vi "Main.vi"() -> ()   [LabVIEW 2018, in "Main.lvlib"]
uses:
  Main.lvlib
  database/Items--cluster.ctl
  database/Purchased_Items--cluster.ctl
  database/Visits--cluster.ctl
  image management/Image Management.lvlib
  receipt parsing/Receipt Parsing.lvlib
  database/Database.lvlib
panel:
  out "Timestamp":timestamp[](array[timestamp])
  out "TotalPrice":dbl
  out "Unit":string[](array[string])
  out "NumberOfUnits":dbl[](array[numeric])
  out "TaxStatus":string[](array[string])
  out "PrintedNames":string[](array[string])
  out "Prices":string[](array[string])
  out "Items":string[](array[string])
  out "Footer":string[](array[string])
  out "Header":string[](array[string])
  out "Main Body":string[](array[string])
  out "Image 2":T1(plugin-control)
  out "Array":string[](array[string])
  out "Columns (Pixels)":i32
  out "Rows (Pixels)":i32
  out "Image":T1(plugin-control)
  out "Rows Where Whitespace Starts":i32[](array[numeric])
  out "Image Pixels (I16)":i16[][](array[numeric])
  out "Error Out":errorcluster
  in  "Error In":errorcluster
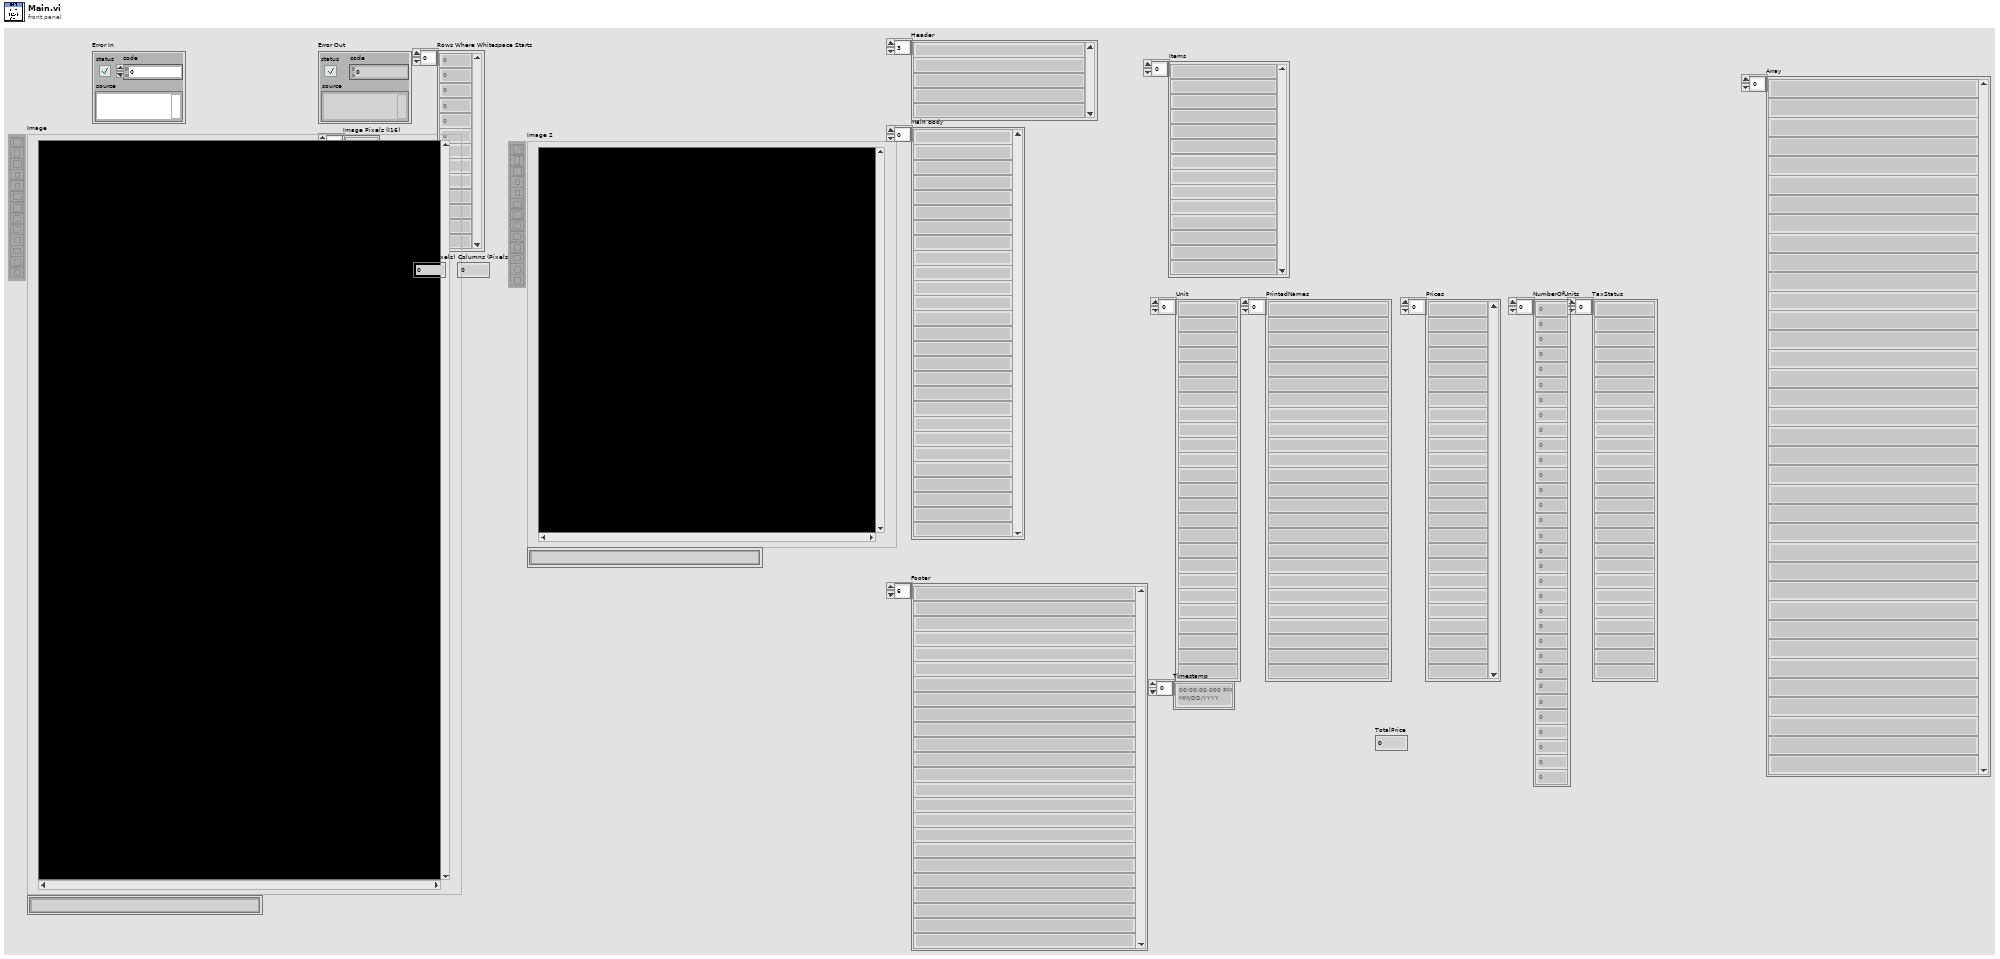
[diagram p1: front panel]
types:
  T1 = typedef "IMAQ Image.ctl" = refnum<image>
  T2 = typedef "Database.lvlib/Visits--cluster.ctl" = cluster{"Timestamp":timestamp, "TotalSpend":dbl, "SpendTaxedA":dbl, "SpendTaxedB":dbl, "Location":string, "NumberOfItems":i32, "NumberOfUniqueItems":i32, "TotalDiscount":dbl}
  T3 = typedef "Database.lvlib/Purchased_Items--cluster.ctl" = cluster{"ItemName":string, "Date":timestamp, "TotalPriceIncludingDiscount":dbl, "NumberOfUnits":i32, "VisitID":i32, "TotalDiscount":dbl}
  T4 = typedef "Database.lvlib/Items--cluster.ctl" = cluster{"ItemName":string, "PrintedNames":string, "TaxStatus":string, "Unit":string, "IsFood":bool, "IsVeg":bool, "IsFavourite":bool}
  T5 = typedef "ROI Descriptor" = cluster{"Global Rectangle":i32[], "Contours":cluster{"ID":enum32{"External", "Internal"}, "Type":u32, "Coordinates":i32[]}[]}
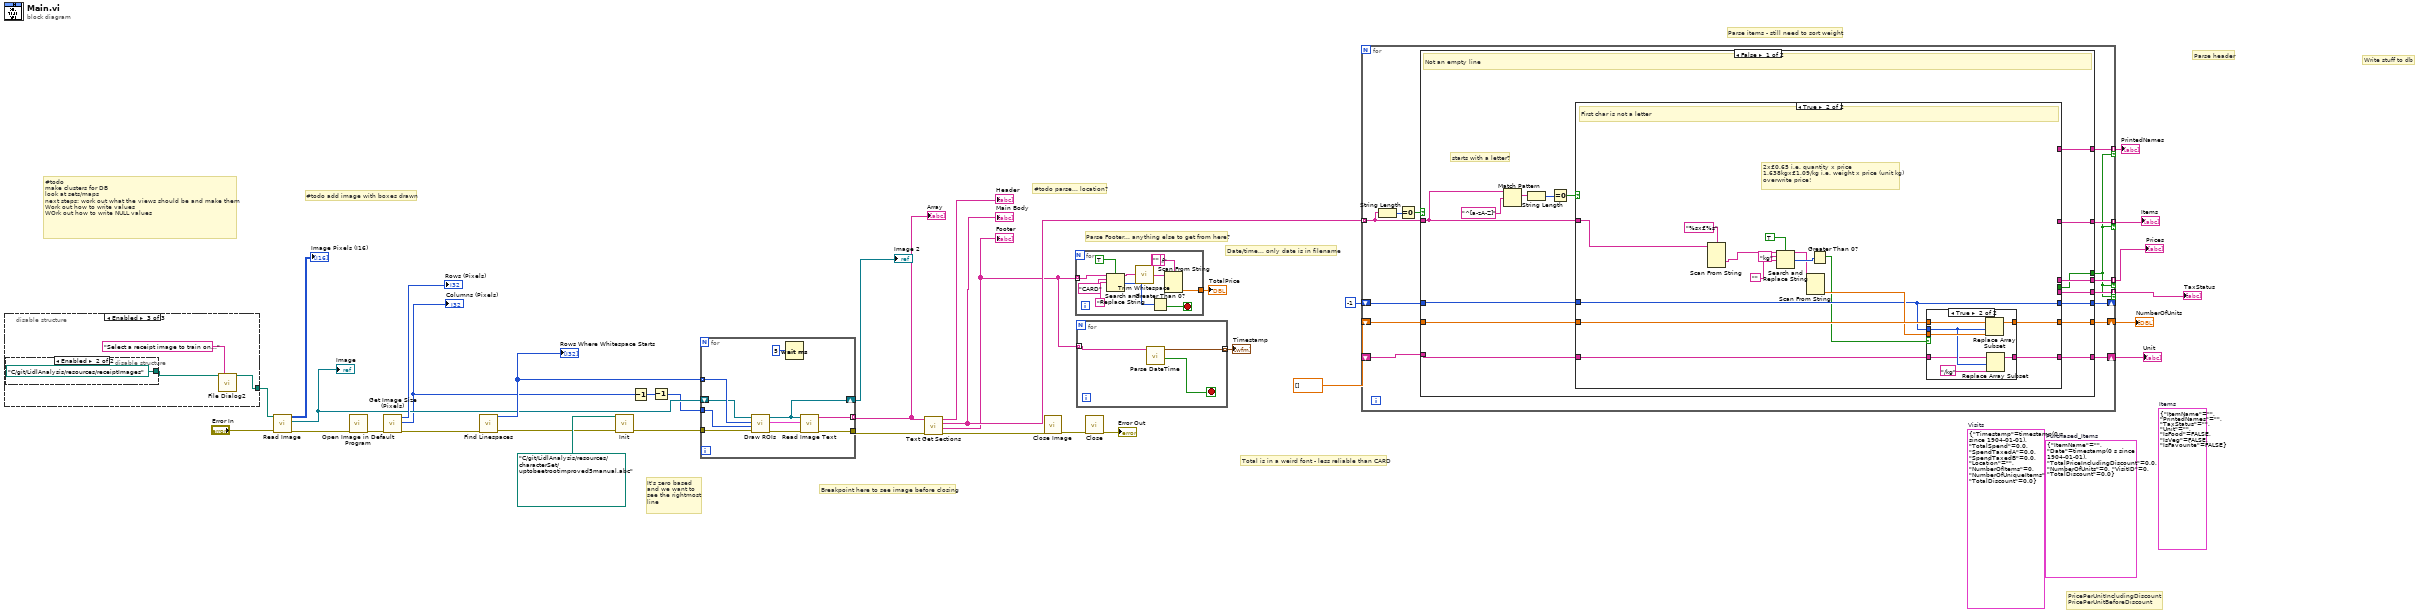
[diagram p0: block diagram]
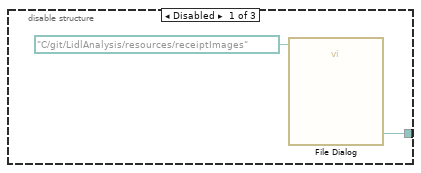
[diagram p2: hidden frame]
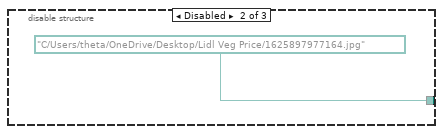
[diagram p3: hidden frame]
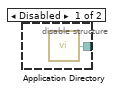
[diagram p4: hidden frame]
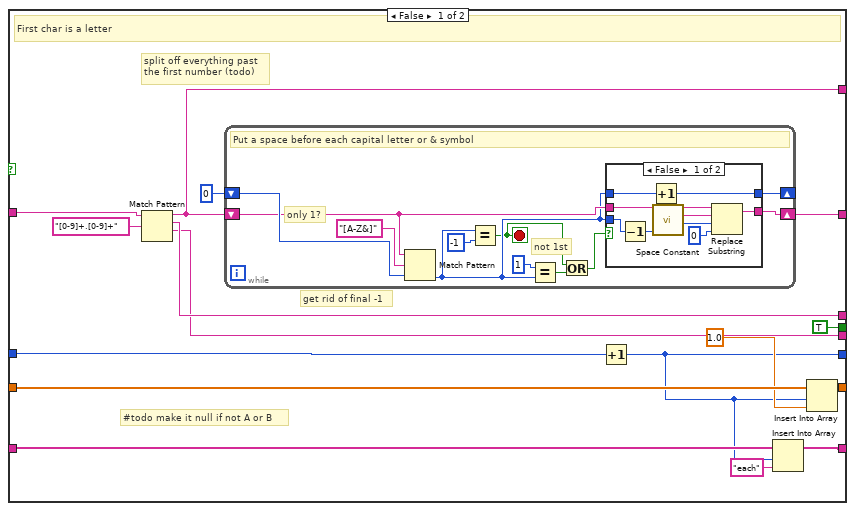
[diagram p5: hidden frame]
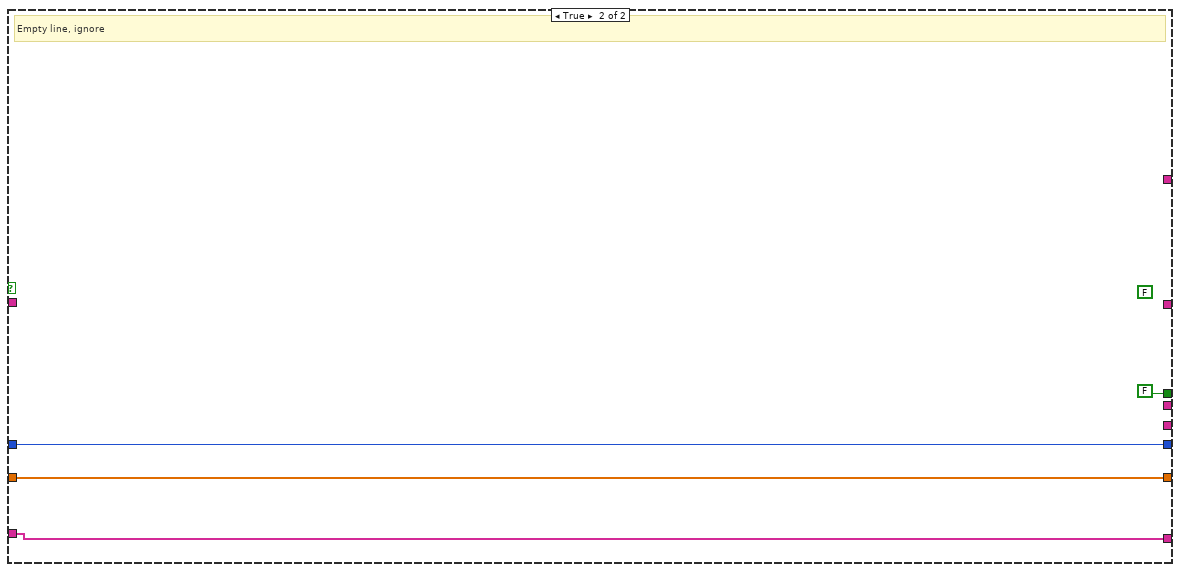
[diagram p8: hidden frame]
diagram:
  (unwired) T2 {"Timestamp"=timestamp(0 s since 1904-01-01), "TotalSpend"=0.0, "SpendTaxedA"=0.0, "SpendTaxedB"=0.0, "Location"="", "NumberOfItems"=0, "NumberOfUniqueItems"=0, "TotalDiscount"=0.0}  # Visits
  (unwired) T3 {"ItemName"="", "Date"=timestamp(0 s since 1904-01-01), "TotalPriceIncludingDiscount"=0.0, "NumberOfUnits"=0, "VisitID"=0, "TotalDiscount"=0.0}  # Purchased_Items
  (unwired) T4 {"ItemName"="", "PrintedNames"="", "TaxStatus"="", "Unit"="", "IsFood"=FALSE, "IsVeg"=FALSE, "IsFavourite"=FALSE}  # Items
  # "Date/time... only date is in filename"
  # "#todo\nmake clusters for DB\nlook at sets/maps\nnext steps: work out what the views should be and make them\nWork out how to write values\nWOrk out how to write NULL values"
  # "#todo parse... location?"
  # "Parse Footer... anything else to get from here?"
  # "Total is in a weird font - less reliable than CARD"
  # "PricePerUnitIncludingDiscount\nPricePerUnitBeforeDiscount"
  # "Write stuff to db"
  # "Parse header"
  # "Parse items - still need to sort weight"
  # "Breakpoint here to see image before closing"
  # "It's zero based\nand we want to\nsee the rightmost\nline"
  # "#todo add image with boxes drawn"
  n1 = disable-structure shown="Enabled" {
    disable-tunnel: [w36 path "C:/Users/theta/OneDrive/Desktop/Lidl Veg Price/1625897977164.jpg" ("File Path") w38] -> w5
    frame Disabled {
      n2 = call "File Dialog"("start path"=path "C:/git/LidlAnalysis/resources/receiptImages") -> ("selected path"=w36:path)  [unwired: 11 in, 3 out]
    }
    frame Disabled {
    }
    frame Enabled {
      n3 = disable-structure shown="Enabled" {
        disable-tunnel: [w41 path "C:/git/LidlAnalysis/resources/receiptImages" ("start path")] -> w39
        frame Disabled {
          n4 = call <vilib>:"Application Directory.vi"() -> ("Application Directory"=w41:path)
        }
        frame Enabled {
        }
      }
      n5 = call "File Dialog2"("start path"=w39, "prompt"="Select a receipt image to train on...") -> ("selected path"=w38:path)  [unwired: 10 in, 3 out]
    }
  }
  n6 = call "Read Image.vi"("Error In"="Error In", "File Path"=w5) -> ("Error Out"=w2:errorcluster, "Image"=w29:T1, "Image Pixels (I16)"=→"Image Pixels (I16)":u8[][])  [unwired: 7 in]
  "Image" <- w29
  n7 = call "Open Image in Default Program.vi"("error in (no error)"=w2) -> ("error out"=w1:errorcluster)  [unwired: 10 in]
  n8 = call "Get Image Size (Pixels).vi"("Error In"=w1) -> ("Error Out"=w32:errorcluster, "Columns (Pixels)"=w28:i32, "Rows (Pixels)"=→"Rows (Pixels)":i32)  [unwired: 8 in]
  "Columns (Pixels)" <- w28
  n9 = call "Find Linespaces.vi"("error in (no error)"=w32) -> ("error out"=w20:errorcluster, "Rows where whitespace starts"=w30:i32[])  [unwired: 9 in]
  "Rows Where Whitespace Starts" <- w30
  n10 = call "Init.vi"("error in (no error)"=w20, "File Path"=path "C:/git/LidlAnalysis/resources/characterSet/uptobeetrootimproved5manual.abc") -> ("error out"=w21:errorcluster)  [unwired: 9 in]
  n11 = Decrement(x=w28) -> (x-1=w27:i32)
  n12 = Decrement(x=w27) -> (x-1=w26:i32)
  n13 = for {
    tunnel: w30 -> [w51] mode=indexing
    tunnel: w26 -> [w52]
    shift-right: [w44] -> w22
    shift-left: w29 -> [w50]
    tunnel: [w48] -> w16
    tunnel: [w47] -> w19 mode=indexing
    tunnel: w21 -> [w46]
    n14 = call "Draw ROIs.vi"("error in (no error)"=w46, "Numeric"=w52, "index of element"=w51, "Refnum in"=w50) -> ("error out"=w45:errorcluster, "ROI Descriptor"=w43:T5, "Refnum out"=w44:T1)  [unwired: 5 in]
    n15 = Wait (ms)(milliseconds to wait=u32 5) -> ()  [unwired: 1 out]
    n16 = call "Read Image Text.vi"("Error In"=w45, "ROI Descriptor"=w43, "Image Ref"=w44) -> ("Error Out"=w48:errorcluster, "Line of Text"=w47:string)  [unwired: 7 in]
  }
  "Array" <- w19
  "Image 2" <- w22
  n17 = call "Text Get Sections.vi"("Error In"=w16, "Receipt Lines"=w19) -> ("Error Out"=w17:errorcluster, "Footer"=w4:string[], "Main Body"=w13:string[], "Header"=→"Header":string[])  [unwired: 6 in]
  "Main Body" <- w13
  "Footer" <- w4
  n18 = call "Close Image.vi"("error in (no error)"=w17) -> ("error out"=w23:errorcluster)  [unwired: 10 in]
  n19 = for {
    tunnel: w4 -> [w62] mode=indexing
    tunnel: [w55] -> w6
    stop <- w54 stop-if-true
    (unwired) "%f" ("format string")
    n20 = Search and Replace String(case sensitive?=TRUE ("ignore case? (F)"), input string=w62, search string="CARD", replace string="") -> (result string=w58:string, number of replacements=w53:i32)  [unwired: 4 in, 2 out]
    n21 = call <vilib>:"Trim Whitespace.vi"("string"=w58) -> ("trimmed string"=w57:string)  [unwired: 1 in]
    n22 = Greater Than 0?(x=w53) -> (x > 0?=w54:bool)
    n23 = Scan From String(format string="", input string=w57) -> (output 1=w55:dbl)  [unwired: 3 in, 3 out]
  }
  "TotalPrice" <- w6
  n24 = for {
    tunnel: w4 -> [w65] mode=indexing
    tunnel: [w63] -> w3 mode=indexing
    stop <- w64 stop-if-true
    n25 = call "Parse DateTime.vi"("Line containing datetime"=w65) -> ("Success?"=w64:bool, "time stamp"=w63:timestamp)  [unwired: 9 in]
  }
  "Timestamp" <- w3
  n26 = call "Close.vi"("error in (no error)"=w23) -> ("error out"=→"Error Out":errorcluster)  [unwired: 10 in]
  n27 = for {
    tunnel: w13 -> [w77] mode=indexing
    tunnel: [w79] -> w15 mode=indexing if=w72
    tunnel: [w78] -> w14 mode=indexing if=w72
    tunnel: [w74] -> w12 mode=indexing if=w72
    tunnel: [w73] -> w11 mode=indexing if=w72
    shift-right: [w71] -> w10
    shift-left: dbl[] [] -> [w70]
    shift-right: [w68] -> _
    shift-left: -1 -> [w69]
    shift-right: [w67] -> w7
    shift-left: _ -> [w66]
    n28 = String Length(string=w77) -> (length=w76:i32)
    n29 = Equal To 0?(x=w76) -> (x = 0?=w75:bool)
    n30 = case shown="False" w75 {
      tunnel: [w95 _] -> w79
      tunnel: [w94 _] -> w78
      tunnel: w77 -> [w89 _]
      tunnel: [w88 FALSE] -> w72
      tunnel: [w87 _] -> w74
      tunnel: [w86 _] -> w73
      tunnel: [w83 w159] -> w71
      tunnel: w70 -> [w82 w159]
      tunnel: w69 -> [w84 w158]
      tunnel: [w85 w158] -> w68
      tunnel: [w81 w157] -> w67
      tunnel: w66 -> [w80 w157]
      frame False {
        # "starts with a letter?"
        # "Not an empty line"
        n31 = Match Pattern(string=w89, regular expression="^[a-zA-Z]") -> (match substring=w90:string)  [unwired: 1 in, 3 out]
        n32 = String Length(string=w90) -> (length=w93:i32)
        n33 = Equal To 0?(x=w93) -> (x = 0?=w92:bool)
        n34 = case shown="True" w92 {
          tunnel: w89 -> [w109 w147]
          tunnel: [w110 _] -> w95
          tunnel: [w107 _] -> w94
          tunnel: [TRUE _] -> w88
          tunnel: [w105 _] -> w87
          tunnel: [w104 _] -> w86
          tunnel: [w97 w136] -> w85
          tunnel: w84 -> [w103 w136]
          tunnel: [w102 w138] -> w83
          tunnel: w82 -> [w101 w139]
          tunnel: [w99 w135] -> w81
          tunnel: w80 -> [w98 w134]
          frame False {
            # "#todo make it null if not A or B"
            # "split off everything past\nthe first number (todo)"
            # "get rid of final -1"
            # "First char is a letter"
            n35 = Match Pattern(string=w109, regular expression="[0-9]+.[0-9]+") -> (before substring=w105:string, match substring=w107:string, after substring=w104:string)  [unwired: 1 in, 1 out]
            n36 = while {
              shift-right: [w117] -> _
              shift-left: 0 ("offset past match") -> [w120]
              shift-right: [w119] -> w110
              shift-left: w105 -> [w118]
              stop <- w113 stop-if-true
              # "not 1st"
              # "only 1?"
              # "Put a space before each capital letter or & symbol"
              n37 = Match Pattern(string=w118, regular expression="[A-Z&]", offset (0)=w120) -> (offset past match=w115:i32)  [unwired: 3 out]
              n38 = Equal?(x=w115, y=-1) -> (x = y?=w113:bool)
              n39 = Equal?(x=1, y=w115) -> (x = y?=w116:bool)
              n40 = Or(x=w113, y=w116) -> (x .or. y?=w114:bool)
              n41 = case shown="False" w114 {
                tunnel: w115 -> [w127 _]
                tunnel: [w129 w132] -> w119
                tunnel: w118 -> [w128 w132]
                tunnel: w115 -> [w124 w131]
                tunnel: [w123 w131] -> w117
                frame False {
                  n42 = Decrement(x=w127) -> (x-1=w126:i32)
                  n43 = Increment(x=w124) -> (x+1=w123:i32)
                  n44 = call <vilib>:"Space Constant.vi"() -> ("String"=w130:string)
                  n45 = Replace Substring(2:0 ("length (len. of substring)"), 3:w126, 4:w130, 5:w128) -> (1:w129:string)  [unwired: 1 out]
                }
                frame True {
                }
              }
            }
            n46 = Increment(x=w103) -> (x+1=w97:i32)
            n47 = Insert Into Array(array=w98, index=w97, new element="each" ("new element/subarray")) -> (w99:string[])
            n48 = Insert Into Array(array=w101, index=w97, new element=1.0) -> (w102:dbl[])
          }
          frame True {
            # "2x£0.65 i.e. quantity x price\n1.638kgx£1.09/kg i.e. weight x price (unit kg)\noverwrite price!"
            # "First char is not a letter"
            n49 = Scan From String(format string="%sx£%s", input string=w147) -> (output 1=w144:string)  [unwired: 5 in, 3 out]
            n50 = Search and Replace String(case sensitive?=TRUE ("ignore case? (F)"), input string=w144, search string="kg", replace string="") -> (result string=w140:string, number of replacements=w142:i32)  [unwired: 4 in, 2 out]
            n51 = Scan From String(input string=w140) -> (output 1=w137:dbl)  [unwired: 4 in, 3 out]
            n52 = Greater Than 0?(x=w142) -> (x > 0?=w133:bool)
            n53 = case shown="True" w133 {
              tunnel: w139 -> [w148 w156]
              tunnel: [w148 w155] -> w138
              tunnel: w137 -> [_ w154]
              tunnel: w136 -> [_ w152]
              tunnel: [w149 w151] -> w135
              tunnel: w134 -> [w149 w150]
              frame False {
              }
              frame True {
                n54 = Replace Array Subset(array=w156, new element=w154, index=w152) -> (w155:dbl[])
                n55 = Replace Array Subset(array=w150, new element="/kg" ("search string"), index=w152) -> (w151:string[])
              }
            }
          }
        }
      }
      frame True {
        (unwired) FALSE
        # "Empty line, ignore"
      }
    }
  }
  "Items" <- w15
  "Prices" <- w14
  "PrintedNames" <- w12
  "TaxStatus" <- w11
  "NumberOfUnits" <- w10
  "Unit" <- w7
